vi "launch daemons.vi"(8 "error in":errorcluster, 10 "daemon confg":T1, 11 "module in":refnum<class "TBM module execution interface.lvclass">) -> (0 "error out":errorcluster, 2 "daemons":refnum<vi>[](array[refnum]), 3 "module out":refnum<class "TBM module execution interface.lvclass">)   [LabVIEW 2013, in "TBM module execution interface.lvclass"]
uses:
  TBM module execution interface.lvclass
  daemon interface.ctl
  <vilib>/NI/Tag Bus/data stream/publisher/publisher.lvclass
  <vilib>/NI/Tag Bus/data stream/subscriber/subscriber.lvclass
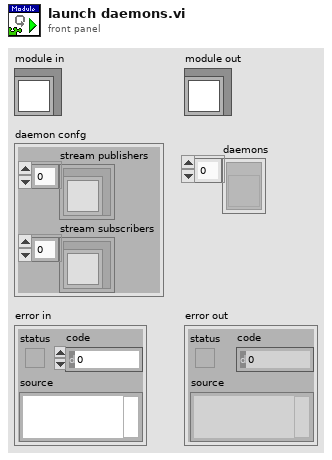
[diagram p1: front panel]
types:
  T1 = typedef "TBM module execution interface.lvclass/daemon interface.ctl" = cluster{"stream publishers":refnum<class "publisher.lvclass">[], "stream subscribers":refnum<class "subscriber.lvclass">[]}
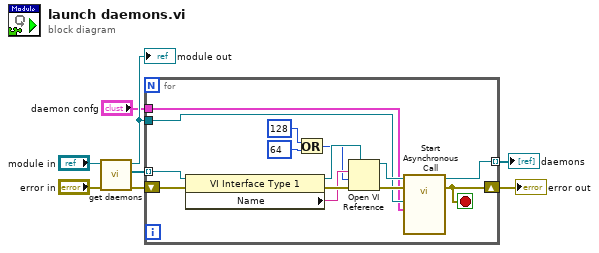
[diagram p0: block diagram]
diagram:
  n1 = call-dynamic "get daemons.vi"("error in"="error in", "module in"="module in") -> ("error out"=w5:errorcluster, "daemons"=w7:refnum<vi>[], "module out"=w3:refnum<class "TBM module execution interface.lvclass">)  [unwired: 7 in]
  "module out" <- w3
  n2 = for {
    tunnel: w7 -> [w22] mode=indexing
    shift-right: [w16] -> w4
    shift-left: w5 -> [w21]
    tunnel: [w14] -> w1 mode=indexing
    tunnel: w3 -> [w10]
    tunnel: "daemon confg" -> [w9]
    stop <- w16 stop-if-true
    n3 = property class="VI Interface Type 1"(reference=w22, error in=w21) -> (reference out=w17:refnum<vi>, error out=w20:errorcluster, "Name"=w18:string)
    n4 = Or(x=128 ("options"), y=64 ("options")) -> (x .or. y?=w12:i32)
    n5 = Open VI Reference(type specifier VI Refnum (for type only)=w17, vi path=w18, options=w12, error in (no error)=w20) -> (vi reference=w15:refnum<vi>, error out=w19:errorcluster)  [unwired: 2 in]
    n6 = call-by-ref "Start Asynchronous Call"(reference=w15, error in=w19, "daemon confg"=w9, "module"=w10) -> (reference out=w14:refnum<vi>, error out=w16:errorcluster)  [unwired: 9 in, 1 out]
  }
  "error out" <- w4
  "daemons" <- w1
